vi "set initial zoom.vi"(9 "reset?":bool, 10 "Image Refs In":T1[](array[typedef]), 11 "DisplayRefsIn(generic class)":refnum<vi>[](array[refnum])) -> ()   [LabVIEW 2017]
doc: "SciScan 1.2 160622"
uses:
  <vilib>/vision/Image Controls.llb/IMAQ Image.ctl
panel:
  out "VI name":string
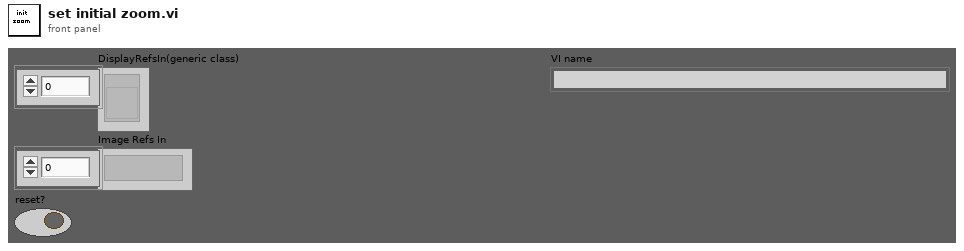
[diagram p1: front panel]
types:
  T1 = typedef "IMAQ Image.ctl" = refnum<image>
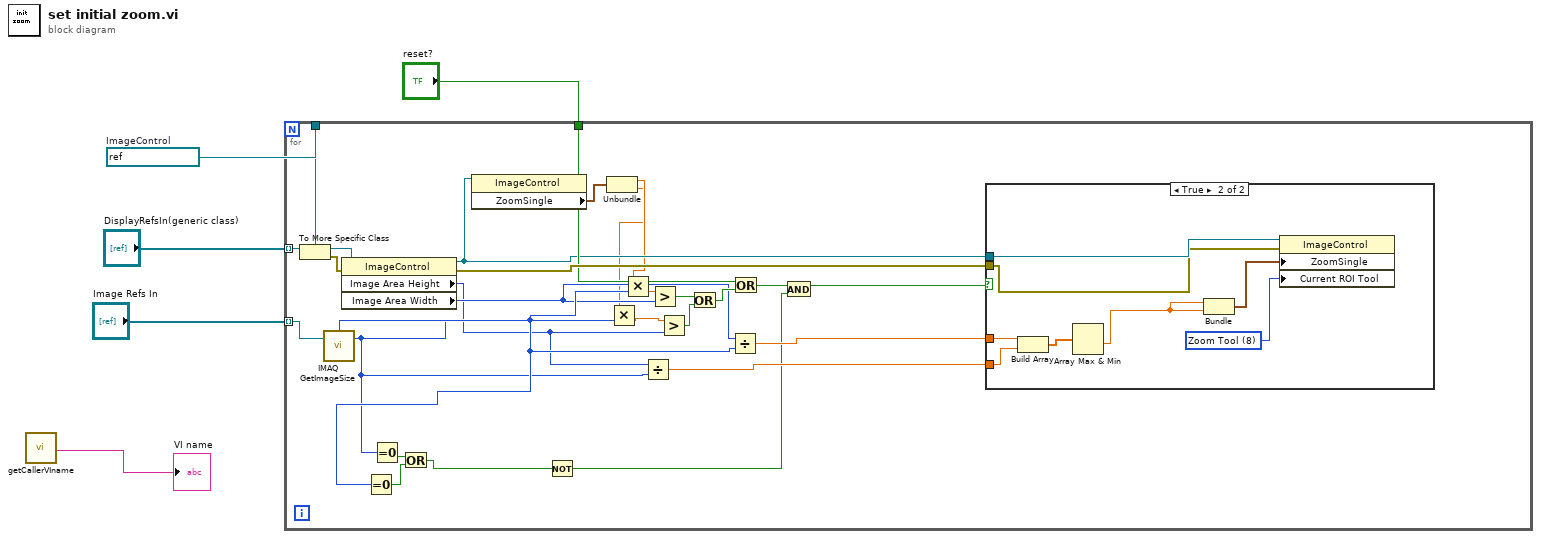
[diagram p0: block diagram]
diagram:
  w5 = refnum<vi> refnum  # ImageControl
  n1 = call "getCallerVIname.vi"() -> ("VI name"=→"VI name":string)  [unwired: 19 in]
  n2 = for {
    tunnel: w5 -> [w33]
    tunnel: "DisplayRefsIn(generic class)" -> [w32] mode=indexing
    tunnel: "Image Refs In" -> [w28] mode=indexing
    tunnel: "reset?" -> [w21]
    n3 = To More Specific Class(target class=w33, reference=w32) -> (specific class reference=w31:refnum<vi>, error out=w29:errorcluster)  [unwired: 1 in]
    n4 = call "IMAQ GetImageSize"("Image"=w28) -> ("Y Resolution"=w14:i32, "X Resolution"=w15:i32)  [unwired: 3 in, 1 out]
    n5 = property class="ImageControl"(reference=w31, error in=w29) -> (reference out=w13:refnum<vi>, error out=w30:errorcluster, "Image Area Height"=w8:u32, "Image Area Width"=w11:u32)
    n6 = Equal To 0?(x=w15) -> (x = 0?=w19:bool)
    n7 = Equal To 0?(x=w14) -> (x = 0?=w20:bool)
    n8 = Or(x=w20, y=w19) -> (x .or. y?=w17:bool)
    n9 = property class="ImageControl"(reference=w13) -> ("ZoomSingle"=w12:cluster{"X":sgl, "Y":sgl})  [unwired: 1 in, 2 out]
    n10 = Not(x=w17) -> (.not. x?=w16:bool)
    n11 = Unbundle(w12) -> ("X"=w9:sgl, "Y"=w6:sgl)
    n12 = Multiply(x=w6, y=w14) -> (x*y=w7:sgl)
    n13 = Multiply(x=w9, y=w15) -> (x*y=w10:sgl)
    n14 = Divide(x=w8, y=w14) -> (x/y=w24:dbl)
    n15 = Greater?(x=w10, y=w11) -> (0:w27:bool)
    n16 = Greater?(x=w7, y=w8) -> (0:w26:bool)
    n17 = Or(x=w27, y=w26) -> (x .or. y?=w25:bool)
    n18 = Divide(x=w11, y=w15) -> (x/y=w23:dbl)
    n19 = Or(x=w21, y=w25) -> (x .or. y?=w22:bool)
    n20 = And(x=w22, y=w16) -> (x .and. y?=w18:bool)
    n21 = case shown="True" w18 {
      tunnel: w13 -> [_ w41]
      tunnel: w30 -> [_ w40]
      tunnel: w24 -> [_ w37]
      tunnel: w23 -> [_ w38]
      frame False {
      }
      frame True {
        w34 = u32 8 items=["Zoom Tool"=8, "Selection Tool"=0, "Pan Tool"=9, "Point Tool"=1, "Line Tool"=2, "Rectangle Tool"=3, "Rotated Rectangle Tool"=12, "Polyline Tool"=10, "Polygon Tool"=5, "Freehand Tool"=11, "Closed Freehand Tool"=6, "Ellipse Tool"=4, "Annulus Tool"=7] ("Current ROI Tool")
        n22 = Build Array(w38, w37) -> (w36:dbl[])
        n23 = Array Max & Min(array=w36) -> (min value=w35:dbl)  [unwired: 3 out]
        n24 = Bundle(w35, w35) -> (w39:cluster{dbl, dbl})  [unwired: 1 in]
        n25 = property class="ImageControl"(reference=w41, error in=w40, "ZoomSingle"=w39, "Current ROI Tool"=w34) -> ()  [unwired: 2 out]
      }
    }
  }
